vi "Pao move.vi"(1 "Color":i32, 2 "Array Position":cluster{"Row":i32, "Column":i32}, 3 "Chess Array":i32[][](array[numeric])=[[140, 130, 120, 110, 100, 111, 121, 131, 141], [-1, -1, -1, -1, -1, -1, -1, -1, -1], [-1, 150, -1, -1, -1, -1, -1, 151, -1], [160, -1, 161, -1, 162, -1, 163, -1, 164], [-1, -1, -1, -1, -1, -1, -1, -1, -1], [-1, -1, -1, -1, -1, -1, -1, -1, -1], [260, -1, 261, -1, 262, -1, 263, -1, 264], [-1, 250, -1, -1, -1, -1, -1, 251, -1], [-1, -1, -1, -1, -1, -1, -1, -1, -1], [240, 230, 220, 210, 200, 211, 221, 231, 241]]) -> (0 "Ju move":cluster{"Row":i32, i32}[](array[cluster]))   [LabVIEW 2009]
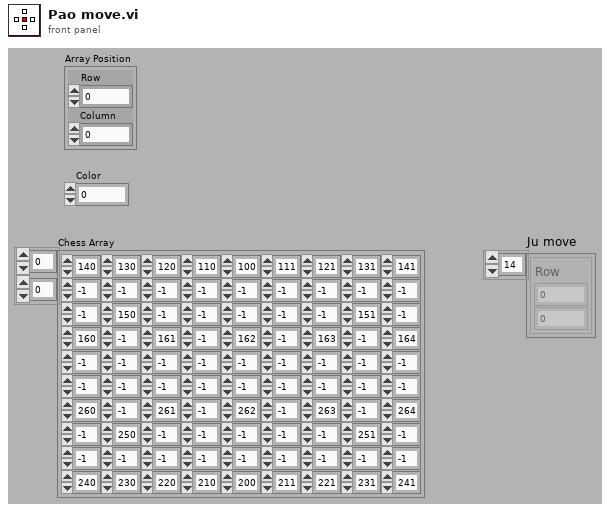
[diagram p1: front panel]
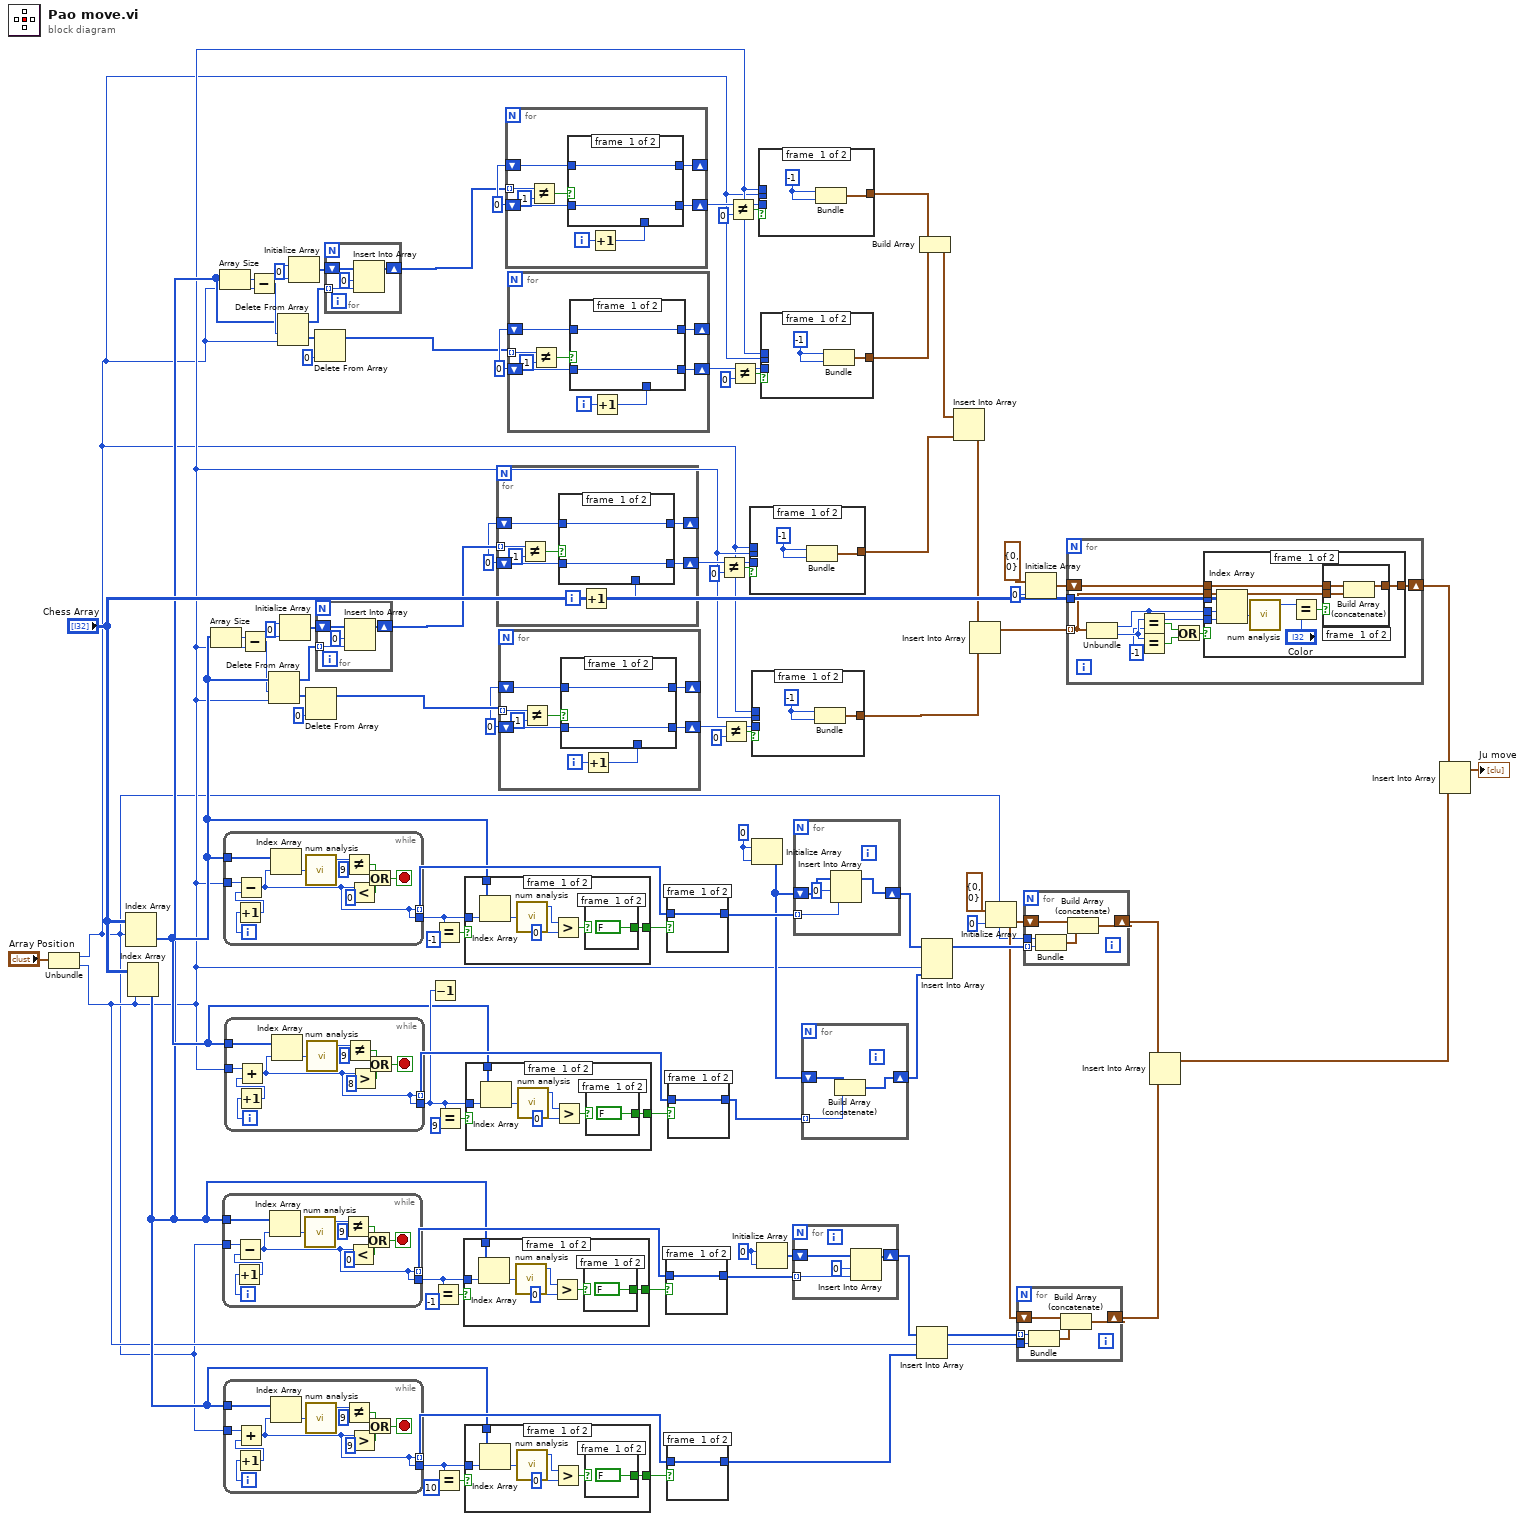
[diagram p0: block diagram]
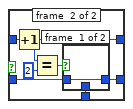
[diagram p4: hidden frame]
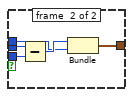
[diagram p6: hidden frame]
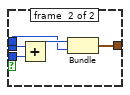
[diagram p7: hidden frame]
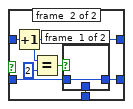
[diagram p8: hidden frame]
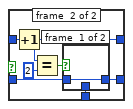
[diagram p10: hidden frame]
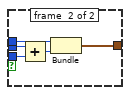
[diagram p12: hidden frame]
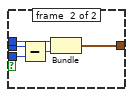
[diagram p13: hidden frame]
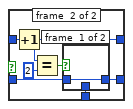
[diagram p14: hidden frame]
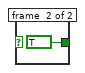
[diagram p16: hidden frame]
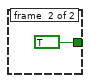
[diagram p17: hidden frame]
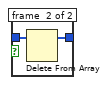
[diagram p18: hidden frame]
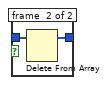
[diagram p19: hidden frame]
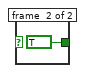
[diagram p20: hidden frame]
diagram:
  w20 = 0 ("Element Data")
  w22 = 0
  w29 = 0
  w34 = 0
  w41 = 0
  w43 = 0 ("Element Data")
  w64 = 0
  w73 = 0 ("Element Data")
  n1 = Unbundle("Array Position") -> ("Row"=w10:i32, "Column"=w11:i32)
  n2 = Index Array(array="Chess Array", index (row)=w10) -> (element=w51:i32[])  [unwired: 1 in]
  n3 = Index Array(array="Chess Array", index (col)=w11) -> (element=w12:i32[])  [unwired: 1 in]
  n4 = Array Size(array=w51) -> (size(s)=w50:i32)
  n5 = Array Size(array=w12) -> (size(s)=w13:i32)
  n6 = while {
    tunnel: w12 -> [w103]
    tunnel: w10 -> [w95]
    tunnel: [w92] -> w67 mode=indexing
    tunnel: [w92] -> w70
    i -> [w94]
    stop <- w98 stop-if-true
    n7 = Increment(x=w94) -> (x+1=w93:i32)
    n8 = Subtract(x=w95, y=w93) -> (x-y=w92:i32)
    n9 = Index Array(array=w103, index=w92) -> (element=w101:i32)
    n10 = call "num analysis.vi"("x"=w101) -> ("Color"=w97:i32)  [unwired: 2 out]
    n11 = Not Equal?(x=w97, y=9) -> (x != y?=w96:bool)
    n12 = Less?(x=w92, y=0) -> (x < y?=w99:bool)
    n13 = Or(x=w96, y=w99) -> (x .or. y?=w98:bool)
  }
  n14 = while {
    tunnel: w51 -> [w115]
    tunnel: w11 -> [w107]
    tunnel: [w104] -> w90 mode=indexing
    tunnel: [w104] -> w53
    i -> [w106]
    stop <- w110 stop-if-true
    n15 = Increment(x=w106) -> (x+1=w105:i32)
    n16 = Subtract(x=w107, y=w105) -> (x-y=w104:i32)
    n17 = Index Array(array=w115, index=w104) -> (element=w113:i32)
    n18 = call "num analysis.vi"("x"=w113) -> ("Color"=w109:i32)  [unwired: 2 out]
    n19 = Not Equal?(x=w109, y=9) -> (x != y?=w108:bool)
    n20 = Less?(x=w104, y=0) -> (x < y?=w111:bool)
    n21 = Or(x=w108, y=w111) -> (x .or. y?=w110:bool)
  }
  n22 = while {
    tunnel: w12 -> [w127]
    tunnel: w10 -> [w119]
    tunnel: [w116] -> w78 mode=indexing
    tunnel: [w116] -> w75
    i -> [w118]
    stop <- w122 stop-if-true
    n23 = Increment(x=w118) -> (x+1=w117:i32)
    n24 = Add(x=w119, y=w117) -> (x+y=w116:i32)
    n25 = Index Array(array=w127, index=w116) -> (element=w125:i32)
    n26 = call "num analysis.vi"("x"=w125) -> ("Color"=w121:i32)  [unwired: 2 out]
    n27 = Not Equal?(x=w121, y=9) -> (x != y?=w120:bool)
    n28 = Greater?(x=w116, y=9) -> (0:w123:bool)
    n29 = Or(x=w120, y=w123) -> (x .or. y?=w122:bool)
  }
  n30 = while {
    tunnel: w51 -> [w139]
    tunnel: w11 -> [w131]
    tunnel: [w128] -> w83 mode=indexing
    tunnel: [w128] -> w52
    i -> [w130]
    stop <- w134 stop-if-true
    n31 = Increment(x=w130) -> (x+1=w129:i32)
    n32 = Add(x=w131, y=w129) -> (x+y=w128:i32)
    n33 = Index Array(array=w139, index=w128) -> (element=w137:i32)
    n34 = call "num analysis.vi"("x"=w137) -> ("Color"=w133:i32)  [unwired: 2 out]
    n35 = Not Equal?(x=w133, y=9) -> (x != y?=w132:bool)
    n36 = Greater?(x=w128, y=8) -> (0:w135:bool)
    n37 = Or(x=w132, y=w135) -> (x .or. y?=w134:bool)
  }
  n38 = Subtract(x=w50, y=w11) -> (x-y=w49:i32)
  n39 = Subtract(x=w13, y=w10) -> (x-y=w14:i32)
  n40 = Delete From Array(array=w51, length=w49, index=w11) -> (deleted portion=w47:i32[], array with subset deleted=w48:i32[])
  n41 = Delete From Array(array=w12, length=w14, index=w10) -> (deleted portion=w16:i32[], array with subset deleted=w15:i32[])
  n42 = Initialize Array(w43, w43) -> (w44:i32[])
  n43 = Initialize Array(w20, w20) -> (w19:i32[])
  n44 = Delete From Array(array=w47, index=0 ("Index")) -> (array with subset deleted=w45:i32[])  [unwired: 1 in, 1 out]
  n45 = Delete From Array(array=w16, index=0 ("Index")) -> (array with subset deleted=w18:i32[])  [unwired: 1 in, 1 out]
  n46 = for {
    tunnel: w48 -> [w141] mode=indexing
    shift-right: [w140] -> w42
    shift-left: w44 -> [w143]
    n47 = Insert Into Array(array=w143, index=0 ("Index"), new element=w141) -> (w140:i32[])
  }
  n48 = for {
    tunnel: w15 -> [w145] mode=indexing
    shift-right: [w144] -> w21
    shift-left: w19 -> [w147]
    n49 = Insert Into Array(array=w147, index=0 ("Index"), new element=w145) -> (w144:i32[])
  }
  n50 = Decrement(x=w52) -> ()  [unwired: 1 out]
  n51 = Equal?(x=w70, y=-1) -> (x = y?=w69:bool)
  n52 = Equal?(x=w53, y=-1) -> (x = y?=w88:bool)
  n53 = Equal?(x=w75, y=10) -> (x = y?=w76:bool)
  n54 = Equal?(x=w52, y=9) -> (x = y?=w85:bool)
  n55 = case shown="False" w69 {
    tunnel: w12 -> [w154 _]
    tunnel: w70 -> [w153 _]
    tunnel: [w149 TRUE] -> w71
    frame #0 {
      n56 = Index Array(array=w154, index=w153) -> (element=w152:i32)
      n57 = call "num analysis.vi"("x"=w152) -> ("Color"=w151:i32)  [unwired: 2 out]
      n58 = Greater?(x=w151, y=0) -> (0:w150:bool)
      n59 = case shown="False" w150 {
        tunnel: [FALSE TRUE] -> w149
        frame #0 {
        }
        frame #1 {
        }
      }
    }
    frame #1 {
    }
  }
  n60 = case shown="False" w88 {
    tunnel: w51 -> [w164 _]
    tunnel: w53 -> [w163 _]
    tunnel: [w159 TRUE] -> w87
    frame #0 {
      n61 = Index Array(array=w164, index=w163) -> (element=w162:i32)
      n62 = call "num analysis.vi"("x"=w162) -> ("Color"=w161:i32)  [unwired: 2 out]
      n63 = Greater?(x=w161, y=0) -> (0:w160:bool)
      n64 = case shown="True" w160 {
        tunnel: [FALSE TRUE] -> w159
        frame #0 {
        }
        frame #1 {
        }
      }
    }
    frame #1 {
    }
  }
  n65 = case shown="False" w76 {
    tunnel: w12 -> [w174 _]
    tunnel: w75 -> [w173 _]
    tunnel: [w169 TRUE] -> w74
    frame #0 {
      n66 = Index Array(array=w174, index=w173) -> (element=w172:i32)
      n67 = call "num analysis.vi"("x"=w172) -> ("Color"=w171:i32)  [unwired: 2 out]
      n68 = Greater?(x=w171, y=0) -> (0:w170:bool)
      n69 = case shown="False" w170 {
        tunnel: [FALSE TRUE] -> w169
        frame #0 {
        }
        frame #1 {
        }
      }
    }
    frame #1 {
    }
  }
  n70 = case shown="False" w85 {
    tunnel: w51 -> [w184 _]
    tunnel: w52 -> [w183 _]
    tunnel: [w179 TRUE] -> w86
    frame #0 {
      n71 = Index Array(array=w184, index=w183) -> (element=w182:i32)
      n72 = call "num analysis.vi"("x"=w182) -> ("Color"=w181:i32)  [unwired: 2 out]
      n73 = Greater?(x=w181, y=0) -> (0:w180:bool)
      n74 = case shown="False" w180 {
        tunnel: [FALSE TRUE] -> w179
        frame #0 {
        }
        frame #1 {
        }
      }
    }
    frame #1 {
    }
  }
  n75 = for {
    tunnel: w42 -> [w196] mode=indexing
    shift-right: [w192] -> _
    shift-left: w41 -> [w193]
    shift-right: [w189] -> w38
    shift-left: w41 -> [w191]
    i -> [w190]
    n76 = Not Equal?(x=w196, y=-1) -> (x != y?=w194:bool)
    n77 = Increment(x=w190) -> (x+1=w188:i32)
    n78 = case shown="True" w194 {
      tunnel: w193 -> [w198 w205]
      tunnel: [w198 w202] -> w192
      tunnel: w191 -> [w197 w201]
      tunnel: w188 -> [_ w200]
      tunnel: [w197 w199] -> w189
      frame #0 {
      }
      frame #1 {
        n79 = Increment(x=w205) -> (x+1=w202:i32)
        n80 = Equal?(x=w202, y=2) -> (x = y?=w204:bool)
        n81 = case shown="True" w204 {
          tunnel: w201 -> [w206 _]
          tunnel: w200 -> [_ w207]
          tunnel: [w206 w207] -> w199
          frame #0 {
          }
          frame #1 {
          }
        }
      }
    }
  }
  n82 = for {
    tunnel: w45 -> [w216] mode=indexing
    shift-right: [w212] -> _
    shift-left: w34 -> [w213]
    shift-right: [w209] -> w37
    shift-left: w34 -> [w211]
    i -> [w210]
    n83 = Not Equal?(x=w216, y=-1) -> (x != y?=w214:bool)
    n84 = Increment(x=w210) -> (x+1=w208:i32)
    n85 = case shown="True" w214 {
      tunnel: w213 -> [w218 w225]
      tunnel: [w218 w222] -> w212
      tunnel: w211 -> [w217 w221]
      tunnel: w208 -> [_ w220]
      tunnel: [w217 w219] -> w209
      frame #0 {
      }
      frame #1 {
        n86 = Increment(x=w225) -> (x+1=w222:i32)
        n87 = Equal?(x=w222, y=2) -> (x = y?=w224:bool)
        n88 = case shown="True" w224 {
          tunnel: w221 -> [w226 _]
          tunnel: w220 -> [_ w227]
          tunnel: [w226 w227] -> w219
          frame #0 {
          }
          frame #1 {
          }
        }
      }
    }
  }
  n89 = for {
    tunnel: w21 -> [w236] mode=indexing
    shift-right: [w232] -> _
    shift-left: w22 -> [w233]
    shift-right: [w229] -> w25
    shift-left: w22 -> [w231]
    i -> [w230]
    n90 = Not Equal?(x=w236, y=-1) -> (x != y?=w234:bool)
    n91 = Increment(x=w230) -> (x+1=w228:i32)
    n92 = case shown="True" w234 {
      tunnel: w233 -> [w238 w245]
      tunnel: [w238 w242] -> w232
      tunnel: w231 -> [w237 w241]
      tunnel: w228 -> [_ w240]
      tunnel: [w237 w239] -> w229
      frame #0 {
      }
      frame #1 {
        n93 = Increment(x=w245) -> (x+1=w242:i32)
        n94 = Equal?(x=w242, y=2) -> (x = y?=w244:bool)
        n95 = case shown="True" w244 {
          tunnel: w241 -> [w246 _]
          tunnel: w240 -> [_ w247]
          tunnel: [w246 w247] -> w239
          frame #0 {
          }
          frame #1 {
          }
        }
      }
    }
  }
  n96 = for {
    tunnel: w18 -> [w256] mode=indexing
    shift-right: [w252] -> _
    shift-left: w29 -> [w253]
    shift-right: [w249] -> w26
    shift-left: w29 -> [w251]
    i -> [w250]
    n97 = Not Equal?(x=w256, y=-1) -> (x != y?=w254:bool)
    n98 = Increment(x=w250) -> (x+1=w248:i32)
    n99 = case shown="True" w254 {
      tunnel: w253 -> [w258 w265]
      tunnel: [w258 w262] -> w252
      tunnel: w251 -> [w257 w261]
      tunnel: w248 -> [_ w260]
      tunnel: [w257 w259] -> w249
      frame #0 {
      }
      frame #1 {
        n100 = Increment(x=w265) -> (x+1=w262:i32)
        n101 = Equal?(x=w262, y=2) -> (x = y?=w264:bool)
        n102 = case shown="True" w264 {
          tunnel: w261 -> [w266 _]
          tunnel: w260 -> [_ w267]
          tunnel: [w266 w267] -> w259
          frame #0 {
          }
          frame #1 {
          }
        }
      }
    }
  }
  n103 = case shown="True" w71 {
    tunnel: w67 -> [w268 w270]
    tunnel: [w268 w269] -> w80
    frame #0 {
    }
    frame #1 {
      n104 = Delete From Array(array=w270) -> (array with subset deleted=w269:i32[])  [unwired: 2 in, 1 out]
    }
  }
  n105 = case shown="True" w87 {
    tunnel: w90 -> [w271 w273]
    tunnel: [w271 w272] -> w81
    frame #0 {
    }
    frame #1 {
      n106 = Delete From Array(array=w273) -> (array with subset deleted=w272:i32[])  [unwired: 2 in, 1 out]
    }
  }
  n107 = case shown="True" w74 {
    tunnel: w78 -> [w274 w276]
    tunnel: [w274 w275] -> w54
    frame #0 {
    }
    frame #1 {
      n108 = Delete From Array(array=w276) -> (array with subset deleted=w275:i32[])  [unwired: 2 in, 1 out]
    }
  }
  n109 = case shown="True" w86 {
    tunnel: w83 -> [w277 w279]
    tunnel: [w277 w278] -> w65
    frame #0 {
    }
    frame #1 {
      n110 = Delete From Array(array=w279) -> (array with subset deleted=w278:i32[])  [unwired: 2 in, 1 out]
    }
  }
  n111 = Not Equal?(x=w38, y=0) -> (x != y?=w39:bool)
  n112 = Not Equal?(x=w37, y=0) -> (x != y?=w36:bool)
  n113 = Not Equal?(x=w25, y=0) -> (x != y?=w24:bool)
  n114 = Not Equal?(x=w26, y=0) -> (x != y?=w27:bool)
  n115 = case shown="False" w39 {
    tunnel: w11 -> [_ w286]
    tunnel: w38 -> [_ w285]
    tunnel: w10 -> [_ w284]
    tunnel: [w281 w282] -> w32
    frame #0 {
      w280 = -1
      n116 = Bundle(w280, w280) -> (w281:cluster{i32, i32})  [unwired: 1 out]
    }
    frame #1 {
      n117 = Subtract(x=w286, y=w285) -> (x-y=w283:i32)
      n118 = Bundle("Row"=w284, w283) -> (w282:cluster{"Row":i32, i32})  [unwired: 1 out]
    }
  }
  n119 = case shown="False" w36 {
    tunnel: w11 -> [_ w293]
    tunnel: w37 -> [_ w292]
    tunnel: w10 -> [_ w291]
    tunnel: [w287 w289] -> w33
    frame #0 {
      w288 = -1
      n120 = Bundle(w288, w288) -> (w287:cluster{i32, i32})  [unwired: 1 out]
    }
    frame #1 {
      n121 = Add(x=w293, y=w292) -> (x+y=w290:i32)
      n122 = Bundle("Row"=w291, w290) -> (w289:cluster{"Row":i32, i32})  [unwired: 1 out]
    }
  }
  n123 = Initialize Array(w64, w64) -> (w63:i32[])
  n124 = Initialize Array(w73, w73) -> (w72:i32[])
  n125 = case shown="True" w24 {
    tunnel: w10 -> [_ w300]
    tunnel: w25 -> [_ w299]
    tunnel: w11 -> [_ w296]
    tunnel: [w295 w298] -> w31
    frame #0 {
      w294 = -1
      n126 = Bundle(w294, w294) -> (w295:cluster{i32, i32})  [unwired: 1 out]
    }
    frame #1 {
      n127 = Subtract(x=w300, y=w299) -> (x-y=w297:i32)
      n128 = Bundle(w297, "Column"=w296) -> (w298:cluster{i32, "Column":i32})  [unwired: 1 out]
    }
  }
  n129 = case shown="True" w27 {
    tunnel: w10 -> [_ w307]
    tunnel: w26 -> [_ w306]
    tunnel: w11 -> [_ w303]
    tunnel: [w301 w305] -> w30
    frame #0 {
      w302 = -1
      n130 = Bundle(w302, w302) -> (w301:cluster{i32, i32})  [unwired: 1 out]
    }
    frame #1 {
      n131 = Add(x=w307, y=w306) -> (x+y=w304:i32)
      n132 = Bundle(w304, "Column"=w303) -> (w305:cluster{i32, "Column":i32})  [unwired: 1 out]
    }
  }
  n133 = for {
    shift-right: [w309] -> w79
    shift-left: w72 -> [w310]
    tunnel: w80 -> [w308] mode=indexing
    n134 = Insert Into Array(array=w310, index=0 ("Index"), new element=w308) -> (w309:i32[])
  }
  n135 = for {
    shift-right: [w314] -> w82
    shift-left: w63 -> [w315]
    tunnel: w81 -> [w313] mode=indexing
    n136 = Insert Into Array(array=w315, index=0 ("Index"), new element=w313) -> (w314:i32[])
  }
  n137 = for {
    tunnel: w65 -> [w317] mode=indexing
    shift-right: [w316] -> w62
    shift-left: w63 -> [w318]
    n138 = Build Array (concatenate)(w318, w317) -> (w316:i32[])
  }
  n139 = Insert Into Array(array=w79, new element=w54) -> (w56:i32[])  [unwired: 1 in]
  n140 = Build Array(w31, w30) -> (w9:cluster{i32, "Column":i32}[])
  n141 = Insert Into Array(array=w82, new element #1=w11, new element #2=w62) -> (w61:i32[])  [unwired: 1 in]
  n142 = Insert Into Array(array=w9, new element=w32) -> (w8:cluster{i32, "Column":i32}[])  [unwired: 1 in]
  n143 = Insert Into Array(array=w8, new element=w33) -> (w7:cluster{i32, "Column":i32}[])  [unwired: 1 in]
  n144 = Initialize Array(cluster{"Row":i32, i32} {"Row"=0, 0} ("Output Cluster"), 0 ("Dimension Size")) -> (w58:cluster{"Row":i32, i32}[])
  n145 = for {
    shift-right: [w321] -> w55
    shift-left: w58 -> [w322]
    tunnel: w56 -> [w320] mode=indexing
    tunnel: w11 -> [w319]
    n146 = Bundle("Element Data"=w320, "Column"=w319) -> (w323:cluster{"Element Data":i32, "Column":i32})  [unwired: 1 out]
    n147 = Build Array (concatenate)(w322, w323) -> (w321:cluster{"Element Data":i32, "Column":i32}[])
  }
  n148 = for {
    tunnel: w10 -> [w328]
    tunnel: w61 -> [w327] mode=indexing
    shift-right: [w324] -> w57
    shift-left: w58 -> [w325]
    n149 = Bundle("Row"=w328, w327) -> (w326:cluster{"Row":i32, i32})  [unwired: 1 out]
    n150 = Build Array (concatenate)(w325, w326) -> (w324:cluster{"Row":i32, i32}[])
  }
  n151 = Initialize Array(cluster{i32, "Column":i32} {0, "Column"=0}, 0 ("Dimension Size")) -> (w4:cluster{i32, "Column":i32}[])
  n152 = for {
    shift-right: [w332] -> w3
    shift-left: w4 -> [w333]
    tunnel: w7 -> [w330] mode=indexing
    tunnel: "Chess Array" -> [w331]
    w336 = -1 ("y")
    n153 = Unbundle(w330) -> (w338:i32, "Column"=w337:i32)
    n154 = Equal?(x=w338, y=w336) -> (x = y?=w335:bool)
    n155 = Equal?(x=w337, y=w336) -> (x = y?=w334:bool)
    n156 = Or(x=w335, y=w334) -> (x .or. y?=w329:bool)
    n157 = case shown="False" w329 {
      tunnel: w333 -> [w341 w353]
      tunnel: [w340 w353] -> w332
      tunnel: w338 -> [w347 _]
      tunnel: w337 -> [w346 _]
      tunnel: w331 -> [w348 _]
      tunnel: w330 -> [w339 _]
      frame #0 {
        n158 = Index Array(array=w348, index (row)=w347, index (col)=w346) -> (element=w345:i32)
        n159 = call "num analysis.vi"("x"=w345) -> ("Color"=w344:i32)  [unwired: 2 out]
        n160 = Equal?(x=w344, y="Color") -> (x = y?=w342:bool)
        n161 = case shown="False" w342 {
          tunnel: w341 -> [w351 w352]
          tunnel: [w349 w352] -> w340
          tunnel: w339 -> [w350 _]
          frame #0 {
            n162 = Build Array (concatenate)(w351, w350) -> (w349:cluster{i32, "Column":i32}[])
          }
          frame #1 {
          }
        }
      }
      frame #1 {
      }
    }
  }
  n163 = Insert Into Array(array=w57, new element=w55) -> (w2:cluster{"Row":i32, i32}[])  [unwired: 1 in]
  n164 = Insert Into Array(array=w3, new element=w2) -> (→"Ju move":cluster{i32, "Column":i32}[])  [unwired: 1 in]
